vi "analyseImage.vi"(8 "error in (no error)":errorcluster, 10 "Array":T1(array[cluster]), 11 "AbsorptionDS in":refnum<class "AbsorptionDS.lvclass">) -> (0 "error out":errorcluster, 3 "AbsorptionDS out":refnum<class "AbsorptionDS.lvclass">)   [LabVIEW 2009, in "Tools.lvlib" / "Imaging.lvlib" / "AbsorptionDS.lvclass"]
uses:
  AbsorptionDS.lvclass
  Filing/FileNeologist/FileNeologist.lvclass
  ImageAnalyser.lvclass
  Filing/FileSystem/FileSystem.lvclass
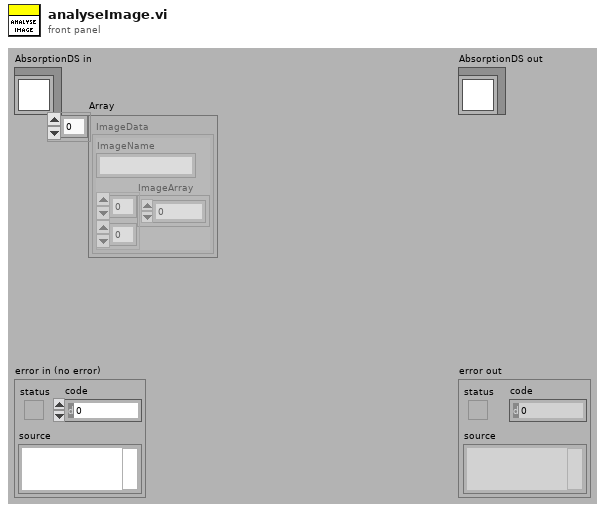
[diagram p1: front panel]
types:
  T1 = cluster{"ImageName":string, "ImageArray":sgl[][]}[]
  T2 = cluster{"Name":string, "Results":dbl[], "AnalysisType":string}
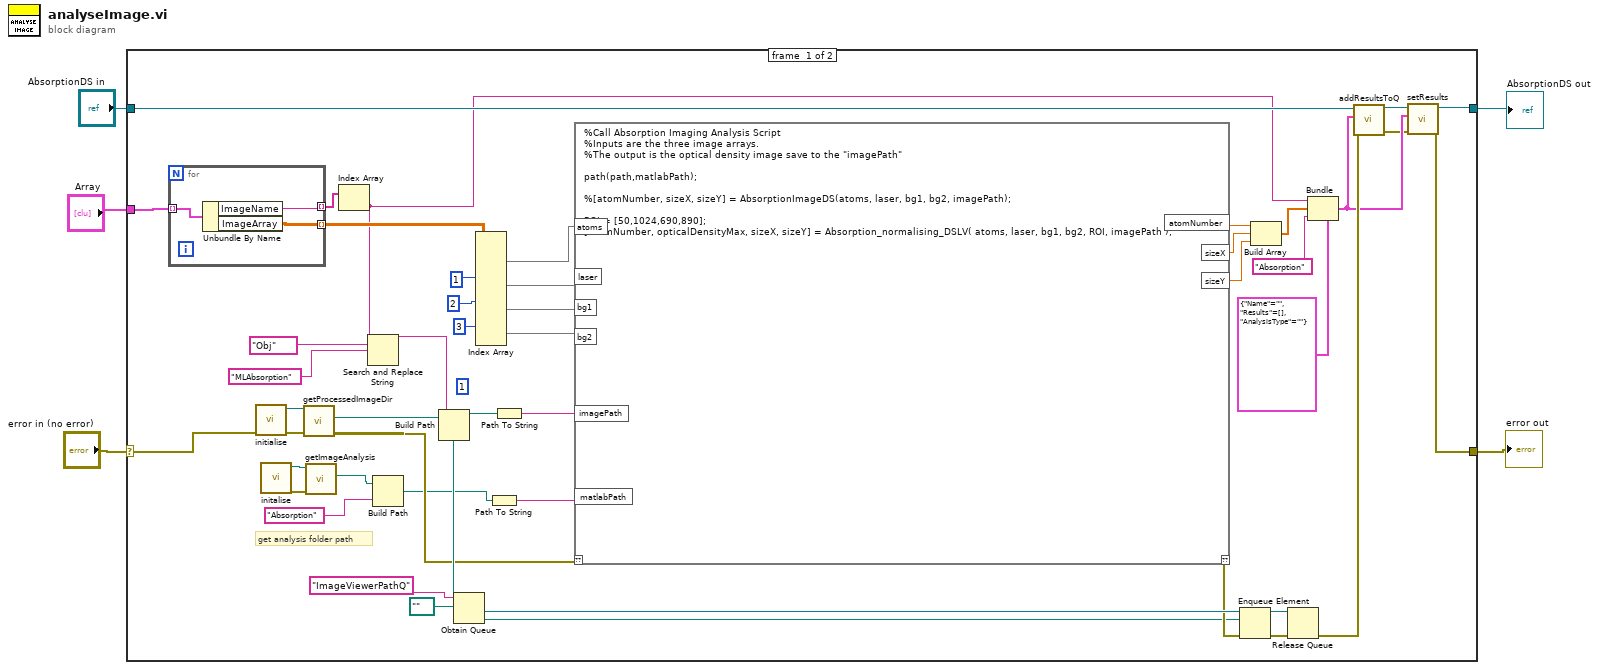
[diagram p0: block diagram]
diagram:
  n1 = case shown="No Error" "error in (no error)" {
    selector: "error in (no error)" -> [w21 w56]
    tunnel: [w9 w56] -> w3
    tunnel: [w12 w55] -> w2
    tunnel: "AbsorptionDS in" -> [w50 w55]
    tunnel: "Array" -> [w49 _]
    frame #0 {
      (unwired) 1
      # "get analysis folder path"
      n2 = for {
        tunnel: w49 -> [w54] mode=indexing
        tunnel: [w53] -> w48 mode=indexing
        tunnel: [w52] -> w44 mode=indexing
        n3 = Unbundle By Name(w54) -> ("ImageName"=w52:string, "ImageArray"=w53:sgl[][])
      }
      n4 = call "initialise.vi"("error in (no error)"=w21) -> ("error out"=w40:errorcluster, "FileNeologist out"=w41:refnum<class "FileNeologist.lvclass">)  [unwired: 9 in]
      n5 = call "initalise.vi"() -> ("error out"=w17:errorcluster, "FileSystem out"=w18:refnum<class "FileSystem.lvclass">)  [unwired: 10 in]
      n6 = call-dynamic "getProcessedImageDir.vi"("error in (no error)"=w40, "FileNeologist in"=w41) -> ("error out"=w20:errorcluster, "Path"=w39:path)  [unwired: 7 in, 1 out]
      n7 = call "getImageAnalysis.vi"("error in (no error)"=w17, "FileSystem in"=w18) -> ("ImageAnalysis"=w16:path)  [unwired: 7 in, 2 out]
      n8 = Index Array(array=w44) -> (element=w24:string)  [unwired: 1 in]
      n9 = Search and Replace String(input string=w24, search string="Obj", replace string="MLAbsorption") -> (result string=w38:string)  [unwired: 5 in, 3 out]
      n10 = Build Path(base path=w16, name or relative path="Absorption") -> (appended path=w14:path)
      n11 = Build Path(base path=w39, name or relative path=w38) -> (appended path=w27:path)
      n12 = Obtain Queue(name (unnamed)="ImageViewerPathQ", element data type=path "") -> (queue out=w35:refnum<queue>)  [unwired: 3 in, 2 out]
      n13 = Index Array(array=w48, index (dim 0) #2=1, index (dim 0) #3=2, index (dim 0) #4=3) -> (element #1=w6:sgl[][], element #2=w46:sgl[][], element #3=w45:sgl[][], element #4=w7:sgl[][])  [unwired: 9 in]
      n14 = Path To String(path=w14) -> (string=w19:string)
      n15 = Path To String(path=w27) -> (string=w32:string)
      n16 = script code="%Call Absorption Imaging Analysis Script \n%Inputs are the three image arrays.\n%The output is the optical density image save to the \"imagePath\"\n\npath(path,matlabPath);\n\n%[atomNumber, sizeX, sizeY] = AbsorptionImageDS(atoms, laser, bg1, bg2, imagePath);\n\nROI = [50,1024,690,890];\n[atomNumber, opticalDensityMax, sizeX, sizeY] = Absorption_normalising_DSLV( atoms, laser, bg1, bg2, ROI, imagePath );"("??"=w20, "bg1"=w45, "laser"=w46, "atoms"=w6, "imagePath"=w32, "matlabPath"=w19, "bg2"=w7) -> ("??"=w28:errorcluster, "atomNumber"=w31:dbl, "sizeX"=w30:dbl, "sizeY"=w29:dbl)
      n17 = Enqueue Element(queue=w35, element=w27, error in (no error)=w28) -> (queue out=w34:refnum<queue>, error out=w33:errorcluster)  [unwired: 1 in, 1 out]
      n18 = Build Array(w31, w30, w29) -> (w25:dbl[])
      n19 = Release Queue(queue=w34, error in (no error)=w33) -> (error out=w26:errorcluster)  [unwired: 1 in, 2 out]
      n20 = Bundle(cluster=T2 {"Name"="", "Results"=[], "AnalysisType"=""} ("output cluster"), "Name"=w24, "Results"=w25, "AnalysisType"="Absorption") -> (w11:T2)
      n21 = call "addResultsToQ.vi"("error in (no error)"=w26, "Results"=w11, "ImageAnalyser in"=w50) -> ("error out"=w10:errorcluster, "ImageAnalyser out"=w13:refnum<class "AbsorptionDS.lvclass">)  [unwired: 7 in]
      n22 = call "setResults.vi"("error in (no error)"=w10, "results"=w11, "ImageAnalyser in"=w13) -> ("error out"=w9:errorcluster, "ImageAnalyser out"=w12:refnum<class "AbsorptionDS.lvclass">)  [unwired: 7 in]
    }
    frame #1 {
    }
  }
  "error out" <- w3
  "AbsorptionDS out" <- w2
